vi "SaveWAVFile.vi"(11 "Old Files":T1[](array[typedef])) -> ()   [LabVIEW 2022 SP3]
uses:
  Curtin1_Label.ctl
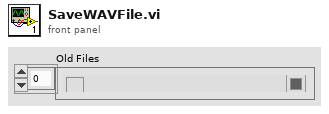
[diagram p1: front panel]
types:
  T1 = typedef "Curtin1_Label.ctl" = cluster{"Show?":bool, "Name":string, "Color":u32, "Path":path, "Show Notes":bool}
  T2 = cluster{"Start freq":dbl, "Hz resolution":dbl, cdb[]}
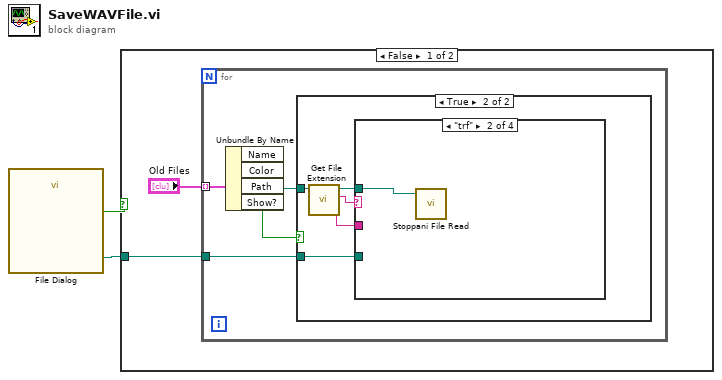
[diagram p0: block diagram]
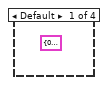
[diagram p3: hidden frame]
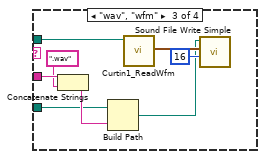
[diagram p4: hidden frame]
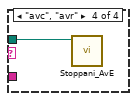
[diagram p5: hidden frame]
diagram:
  n1 = call "File Dialog"() -> ("selected path"=w2:path, "cancelled"=w1:bool)  [unwired: 12 in, 2 out]
  n2 = case shown="False" w1 {
    tunnel: w2 -> [w3 _]
    frame False {
      n3 = for {
        tunnel: "Old Files" -> [w7] mode=indexing
        tunnel: w3 -> [w5]
        n4 = Unbundle By Name(w7) -> ("Path"=w8:path, "Show?"=w6:bool)  [unwired: 2 out]
        n5 = case shown="True" w6 {
          tunnel: w8 -> [_ w11]
          tunnel: w5 -> [_ w9]
          frame False {
          }
          frame True {
            n6 = call <vilib>:"Get File Extension.vi"("file"=w11) -> ("filename without extension"=w10:string, "lowercase file extension"=w12:string, "dup file"=w13:path)  [unwired: 6 in, 2 out]
            n7 = case shown="\"trf\"" w12 {
              tunnel: w13 -> [_ w14 w18 w23]
              tunnel: w10 -> [_ _ w20 _]
              tunnel: w9 -> [_ _ w16 _]
              frame Default {
                (unwired) T2 {"Start freq"=0.0, "Hz resolution"=0.0, []} ("Waveform Graph")
              }
              frame "trf" {
                n8 = call "Stoppani File Read.vi"("String in"=w14) -> ()  [unwired: 2 in, 4 out]
              }
              frame "wav", "wfm" {
                n9 = Concatenate Strings(w20, ".wav" ("string")) -> (w17:string)
                n10 = Build Path(base path=w16, name or relative path=w17) -> (appended path=w15:path)
                n11 = call "Curtin1_ReadWfm.vi"("appended path"=w18) -> ("all waveforms in record"=w22:waveform(dbl)[])  [unwired: 9 in, 1 out]
                n12 = call <vilib>:"Sound File Write Simple.vi"("bits per sample"=16, "data"=w22, "path"=w15) -> ()  [unwired: 7 in, 2 out]
              }
              frame "avc", "avr" {
                n13 = call "Stoppani_AvE.vi"("file (use dialog)"=w23) -> ()  [unwired: 7 in, 4 out]
              }
            }
          }
        }
      }
    }
    frame True {
    }
  }
